vi "GetMfgDateCode.vi"(6 "error in (no error)":errorcluster) -> (0 "error out":errorcluster, 1 "WWYY":string, 2 "Year.Month.Date":string, 3 "WeekYearCode":string)   [LabVIEW 2024]
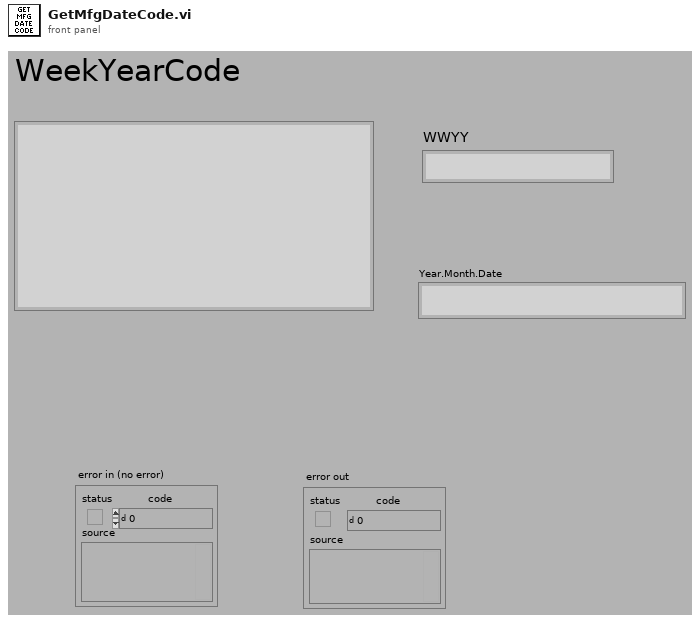
[diagram p1: front panel]
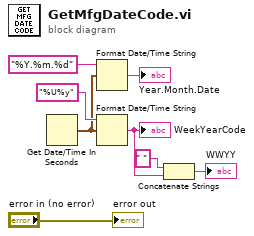
[diagram p0: block diagram]
diagram:
  n1 = Get Date/Time In Seconds() -> (seconds since 1Jan1904=w3:timestamp)
  n2 = Format Date/Time String(time format string (%c)="%Y.%m.%d", seconds (now)=w3) -> (date/time string=→"Year.Month.Date":string)  [unwired: 1 in]
  n3 = Format Date/Time String(time format string (%c)="%U%y", seconds (now)=w3) -> (date/time string=w5:string)  [unwired: 1 in]
  "WeekYearCode" <- w5
  n4 = Concatenate Strings(" " ("string"), w5) -> (→"WWYY":string)
  "error out" <- "error in (no error)"
